vi "Get SICK Data.vi"(8 "error in":errorcluster, 11 "FPGA_MAIN ref in":T2) -> (0 "error out":errorcluster, 1 "Buffer Not Empty":bool, 2 "SICK Data":T1, 3 "FPGA_MAIN ref out":T2)   [LabVIEW 2009]
uses:
  TypeDefs/Sensor TypeDefs/FPGA Main ref.ctl
  TypeDefs/Sensor TypeDefs/SICK Array.ctl
  <vilib>/rvi/interface/nirviMethod/nirviMethod.xnode
  FPGA Bitfiles/Q_IGVC_2010.lvproj_FPGA Target_FPGA_MAIN.vi.lvbitx
  <vilib>/rvi/interface/common/niFpgaNodeNameForErrorReporting.ctl
  <vilib>/rvi/errors/niLvFpgaWhatHappensToTopLevelVI.ctl
  <vilib>/Utility/error.llb/Error Cluster From Error Code.vi
  <vilib>/rvi/errors/niLvFpgaAdjustHostInterfaceError.vi
  <vilib>/LabVIEW Targets/FPGA/RIO/nirio_HostInterface/nirio_WaitOnIRQ.vi
  <vilib>/RVI Host/nirviSupport.llb/nirviErrorClusterFromErrorCode.vi
  NiRioSrv.dll
panel:
  out "Part 4 time":u32
  out "Part 3 time":u32
  out "Part 2 time":u32
  out "Part 1 time":u32
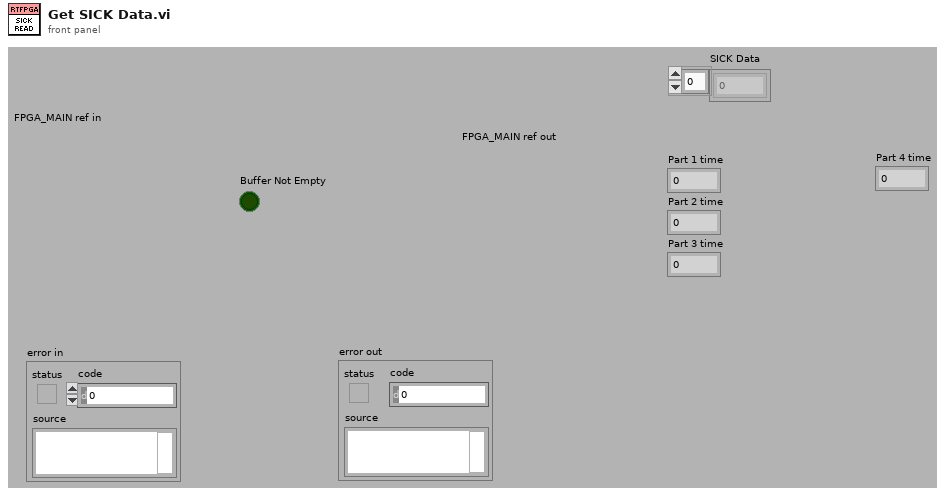
[diagram p1: front panel]
types:
  T1 = typedef "SICK Array.ctl" = u16[]
  T2 = typedef "FPGA Main ref.ctl" = refnum<k20>
  T3 = typedef "niFpgaNodeNameForErrorReporting.ctl" = enum16{"Open FPGA VI Reference", "Read/Write Control", "Invoke Method: Abort", "Invoke Method: Acknowledge IRQ", "Invoke Method: Download", "Invoke Method: FIFO.Configure", "Invoke Method: FIFO.Read", "Invoke Method: FIFO.Start", "Invoke Method: FIFO.Stop", "Invoke Method: FIFO.Write", "Invoke Method: Reset", "Invoke Method: Run", "Invoke Method: Wait on IRQ", "Close FPGA VI Reference"}
  T4 = typedef "niLvFpgaWhatHappensToTopLevelVI.ctl" = enum16{"top level VI scripted behind XNode", "top level VI inlined behind XNode"}
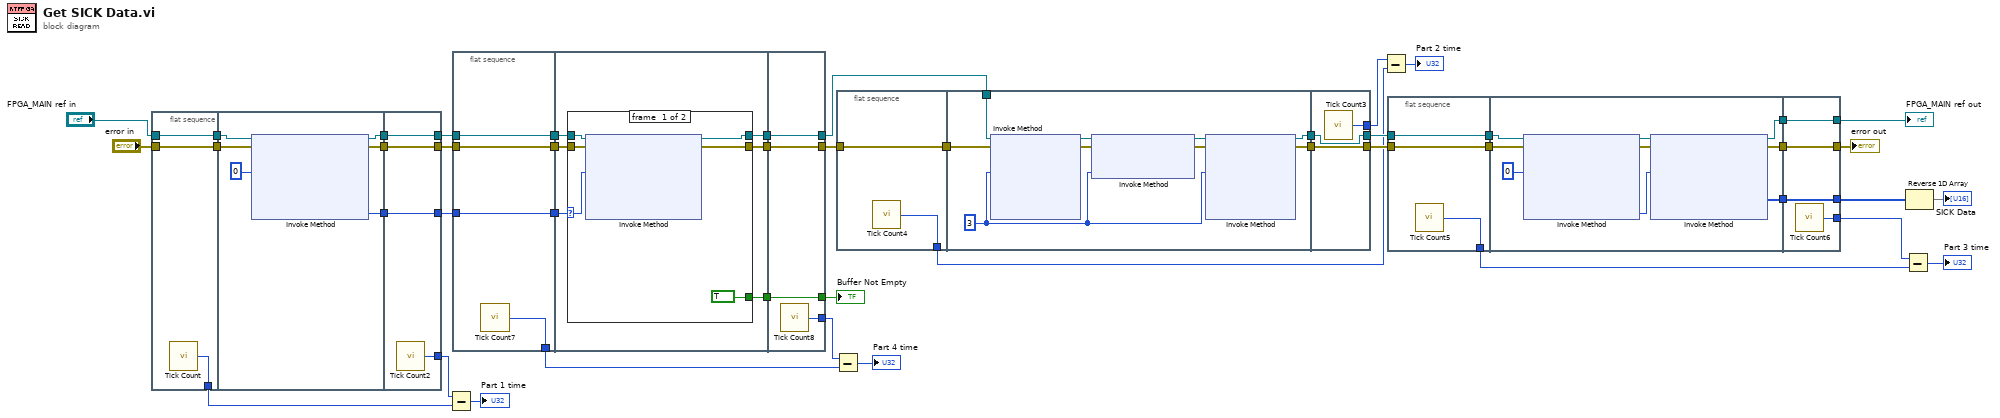
[diagram p0: block diagram]
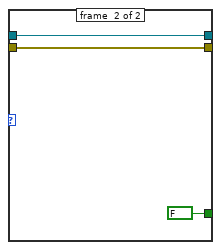
[diagram p2: hidden frame]
diagram:
  n1 = flat-sequence {
    tunnel: "error in" -> [w47]
    tunnel: "FPGA_MAIN ref in" -> [w48]
    tunnel: [w48] -> w32
    tunnel: [w47] -> w31
    tunnel: [w46] -> w26
    tunnel: w32 -> [w50]
    tunnel: w31 -> [w49]
    tunnel: [w53] -> w30
    tunnel: [w52] -> w29
    tunnel: [w51] -> w28
    tunnel: [w128] -> w40
    tunnel: [w129] -> w41
    tunnel: [w130] -> w42
    tunnel: w30 -> [w130]
    tunnel: w29 -> [w129]
    tunnel: w28 -> [w128]
    tunnel: [w127] -> w27
    frame #0 {
      n2 = call "Tick Count"() -> ("Tick Count(uSec)"=w46:u32)
    }
    frame #1 {
      n3 = xnode "Invoke Method"("FPGA VI Reference In"=w50, "error in"=w49, "Number of Elements"=u32 0) -> ("FPGA VI Reference Out"=w52:T2, "error out"=w51:errorcluster, "Elements Remaining"=w53:u32)  [unwired: 1 in, 1 out]
    }
    frame #2 {
      n4 = call "Tick Count2"() -> ("Tick Count(uSec)"=w127:u32)
    }
  }
  n5 = Subtract(x=w27, y=w26) -> (x-y=→"Part 1 time":u32)
  n6 = flat-sequence {
    tunnel: w40 -> [w132]
    tunnel: w41 -> [w133]
    tunnel: w42 -> [w134]
    tunnel: [w134] -> w10
    tunnel: [w133] -> w9
    tunnel: [w132] -> w8
    tunnel: [w131] -> w2
    tunnel: w10 -> [w140]
    tunnel: w9 -> [w139]
    tunnel: w8 -> [w138]
    tunnel: [w137] -> w7
    tunnel: [w136] -> w6
    tunnel: [w135] -> w5
    tunnel: [w223] -> w35
    tunnel: [w224] -> w36
    tunnel: [w225] -> w37
    tunnel: w7 -> [w225]
    tunnel: w6 -> [w224]
    tunnel: w5 -> [w223]
    tunnel: [w222] -> w3
    frame #0 {
      n7 = call "Tick Count7"() -> ("Tick Count(uSec)"=w131:u32)
    }
    frame #1 {
      n8 = case shown="Default" w140 {
        selector: w140 -> [w146 _]
        tunnel: w139 -> [w145 w221]
        tunnel: w138 -> [w144 w220]
        tunnel: [w143 w221] -> w137
        tunnel: [w142 w220] -> w136
        tunnel: [TRUE ("Boolean") FALSE ("Boolean")] -> w135
        frame #0 {
          n9 = xnode "Invoke Method"("FPGA VI Reference In"=w145, "error in"=w144, "Number of Elements"=w146) -> ("FPGA VI Reference Out"=w143:T2, "error out"=w142:errorcluster)  [unwired: 1 in, 2 out]
        }
        frame #1 {
        }
      }
    }
    frame #2 {
      n10 = call "Tick Count8"() -> ("Tick Count(uSec)"=w222:u32)
    }
  }
  n11 = Subtract(x=w3, y=w2) -> (x-y=→"Part 4 time":u32)
  n12 = flat-sequence {
    tunnel: w36 -> [w227]
    tunnel: [w227] -> w24
    tunnel: [w226] -> w19
    tunnel: w37 -> [w231]
    tunnel: w24 -> [w230]
    tunnel: [w229] -> w23
    tunnel: [w228] -> w22
    tunnel: [w547] -> w33
    tunnel: [w548] -> w34
    tunnel: w23 -> [w548]
    tunnel: w22 -> [w547]
    tunnel: [w546] -> w20
    frame #0 {
      n13 = call "Tick Count4"() -> ("Tick Count(uSec)"=w226:u32)
    }
    frame #1 {
      w232 = 3 ("IRQ Number(s)")
      n14 = xnode "Invoke Method"("FPGA VI Reference In"=w231, "error in"=w230, "IRQ Number(s)"=w232) -> ("FPGA VI Reference Out"=w236:T2, "error out"=w235:errorcluster)  [unwired: 1 in, 2 out]
      n15 = xnode "Invoke Method"("FPGA VI Reference In"=w236, "error in"=w235, "IRQ Number(s)"=w232) -> ("FPGA VI Reference Out"=w234:T2, "error out"=w233:errorcluster)
      n16 = xnode "Invoke Method"("FPGA VI Reference In"=w234, "error in"=w233, "IRQ Number(s)"=w232) -> ("FPGA VI Reference Out"=w229:T2, "error out"=w228:errorcluster)  [unwired: 1 in, 2 out]
    }
    frame #2 {
      n17 = call "Tick Count3"() -> ("Tick Count(uSec)"=w546:u32)
    }
  }
  n18 = Subtract(x=w20, y=w19) -> (x-y=→"Part 2 time":u32)
  n19 = flat-sequence {
    tunnel: w33 -> [w550]
    tunnel: w34 -> [w551]
    tunnel: [w551] -> w18
    tunnel: [w550] -> w17
    tunnel: [w549] -> w11
    tunnel: w18 -> [w555]
    tunnel: w17 -> [w554]
    tunnel: [w560] -> w16
    tunnel: [w559] -> w15
    tunnel: [w558] -> w14
    tunnel: [w706] -> w43
    tunnel: [w707] -> w44
    tunnel: [w708] -> w45
    tunnel: w16 -> [w708]
    tunnel: w15 -> [w707]
    tunnel: w14 -> [w706]
    tunnel: [w705] -> w12
    frame #0 {
      n20 = call "Tick Count5"() -> ("Tick Count(uSec)"=w549:u32)
    }
    frame #1 {
      n21 = xnode "Invoke Method"("FPGA VI Reference In"=w555, "error in"=w554, "Number of Elements"=u32 0) -> ("FPGA VI Reference Out"=w552:T2, "error out"=w553:errorcluster, "Elements Remaining"=w557:u32)  [unwired: 1 in, 1 out]
      n22 = xnode "Invoke Method"("FPGA VI Reference In"=w552, "error in"=w553, "Number of Elements"=w557) -> ("FPGA VI Reference Out"=w559:T2, "error out"=w560:errorcluster, "Data"=w558:u16[])  [unwired: 1 in, 1 out]
    }
    frame #2 {
      n23 = call "Tick Count6"() -> ("Tick Count(uSec)"=w705:u32)
    }
  }
  n24 = Subtract(x=w12, y=w11) -> (x-y=→"Part 3 time":u32)
  n25 = Reverse 1D Array(array=w43) -> (reversed array=→"SICK Data":u16[])
  "FPGA_MAIN ref out" <- w44
  "error out" <- w45
  "Buffer Not Empty" <- w35
